vi "pakistan.vi"() -> ()   [LabVIEW 2011]
uses:
  VisualStudio/linking/Debug/linking.dll
panel:
  out "X^2 + Y^2":dbl
  in  "X":dbl
  in  "Y":dbl
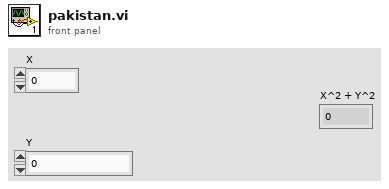
[diagram p1: front panel]
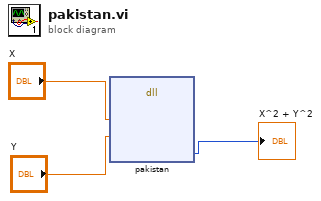
[diagram p0: block diagram]
diagram:
  n1 = dll-call lib="C:/Users/umfehr44.ENG/Desktop/Micromirror Project/GloryofPakistan/VisualStudio/linking/Debug/linking.dll" fn="pakistan"("x"="X", "y"="Y") -> ("z"=→"X^2 + Y^2":i32)  [unwired: 7 in, 2 out]
